vi "Analog Scan.vi"() -> ()   [LabVIEW 2020]
uses:
  Serial Support VISA.llb/Serial Actions.ctl
panel:
  out "He3/He4":dbl=0.027017159547280026 format="%.3f"
  out "Update":bool
  out "Total Pressure":dbl=1.3867864864864864e-05 format="%.3e"
  in  "stop":bool
  out "?":dbl[](graph)=[6.383227176220806e-09, 5.799363057324841e-09, 6.292993630573249e-09, 1.071751592356688e-07, 2.781942675159236e-07, 2.2762632696390657e-07, 3.148853503184713e-07, 4.156592356687898e-07, 5.076602972399151e-07, 5.451220806794055e-07, 5.554108280254777e-07, 5.598842887473461e-07, 4.985690021231423e-07, 3.8966985138004246e-07, 2.408577494692144e-07, 6.305732484076434e-08, 1.80552016985138e-08, 7.371549893842887e-09, 4.512738853503184e-09, 1.0222929936305733e-09, 3.142250530785562e-10, -1.8397027600849257e-09, 1.2845010615711252e-09, 8.70488322717622e-11, 2.2123142250530784e-09, 1.4118895966029723e-09, 4.543524416135881e-10, 5.165605095541402e-09, 8.238853503184713e-09, 1.0167728237791932e-08, 1.1630573248407643e-08, 1.0235668789808917e-08, 1.1387473460721868e-08, 9.991507430997877e-09, 5.780254777070063e-09, 1.959660297239915e-09, -9.851380042462845e-10, 3.7261146496815285e-10, -1.3237791932059447e-09, -5.6263269639065816e-11, -5.679405520169851e-10, -2.227176220806794e-09, 1.0042462845010616e-09, 8.938428874734607e-10, 7.91932059447983e-10, 4.447983014861995e-10, -1.4904458598726114e-09, 2.8662420382165604e-11, 2.083864118895966e-09, -3.5244161358811037e-10, -6.295116772823779e-10, -1.898089171974522e-09, 4.5010615711252653e-10, 1.9479830148619957e-09, -2.210191082802548e-09, 1.7908704883227175e-09, -6.114649681528662e-10, 7.027600849256899e-10, 2.2154989384288745e-09, -2.2367303609341826e-09, 3.5138004246284497e-10, -1.6475583864118898e-09, -1.2420382165605095e-09, 1.8004246284501061e-09, -2.4532908704883226e-09, -4.670912951167728e-11, -2.91932059447983e-10, 1.2738853503184715e-11, 2.489384288747346e-09, -2.265392781316348e-09, 8.439490445859872e-10, -3.354564755838641e-10, -7.526539278131635e-10, 2.421443736730361e-09, -2.700636942675159e-09, 9.861995753715497e-10, -7.887473460721868e-10, -6.157112526539278e-11, 2.832271762208068e-09, -2.252653927813163e-09, 2.62208067940552e-10, 2.1231422505307854e-11, -9.002123142250531e-10, 2.468152866242038e-09, -3.5360934182590233e-09, 8.386411889596603e-10, -5.870488322717621e-10, -3.927813163481953e-11, 2.1687898089171975e-09, -2.6104033970276008e-09, 7.282377919320594e-10, -6.900212314225053e-11, -1.2983014861995753e-09, 1.3832271762208068e-09, -2.6008492569002124e-09, 2.6751592356687895e-10, -5.870488322717621e-10, -2.7388535031847135e-10, 1.8630573248407644e-09, -2.178343949044586e-09, 8.397027600849257e-10, 4.978768577494691e-10, -2.218683651804671e-10, 1.7070063694267515e-09, -1.96072186836518e-09, 3.90552016985138e-09, 5.8046709129511675e-09, 6.473460721868365e-09, 9.766454352441613e-09, 9.27176220806794e-09, 1.16932059447983e-08, 1.3043524416135881e-08, 9.373673036093419e-09, 8.456475583864119e-09, 6.231422505307855e-10, 1.718683651804671e-09, 1.1464968152866242e-10, 1.3322717622080678e-09, 3.2547770700636943e-09, 1.054140127388535e-09, 4.818471337579618e-09, 4.9808917197452225e-09, 3.5e-09, 7.670912951167728e-09, 1.2777070063694267e-08, 5.751273885350318e-08, 1.5892462845010614e-07, 2.25776008492569e-07, 2.7426857749469213e-07, 3.0801380042462845e-07, 3.070297239915074e-07, 2.9790233545647557e-07, 2.338673036093418e-07, 1.5005626326963905e-07, 4.046815286624204e-08, 1.6974522292993628e-08, 1.4698513800424627e-08, 1.4262208067940551e-08, 1.869532908704883e-08, 1.897452229299363e-08, 2.06104033970276e-08, 2.2679405520169852e-08, 1.8743099787685772e-08, 1.7830148619957538e-08, 1.4470276008492568e-08, 3.696072186836518e-08, 8.625265392781315e-08, 1.211496815286624e-07, 1.4909235668789808e-07, 1.649692144373673e-07, 1.6709235668789808e-07, 1.6360828025477706e-07, 1.2956581740976644e-07, 8.94384288747346e-08, 4.8571125265392775e-08, 1.1504458598726114e-07, 2.6974734607218685e-07, 3.562579617834395e-07, 4.158556263269639e-07, 4.545021231422505e-07, 4.449851380042463e-07, 4.240583864118896e-07, 3.339023354564756e-07, 2.2270276008492568e-07, 1.6168895966029725e-07, 5.474246284501061e-07, 1.1831061571125264e-06, 1.4687940552016984e-06, 1.6797356687898089e-06, 1.7986709129511676e-06, 1.7556889596602972e-06, 1.5903195329087047e-06, 1.2338619957537154e-06, 6.22692144373673e-07, 7.33864118895966e-08, 2.1935244161358813e-08, 1.1503184713375797e-08, 4.5902335456475585e-09, 6.038216560509554e-09, 3.182590233545647e-09, 5.26963906581741e-09, 6.270700636942675e-09, 1.559447983014862e-09, 4.739915074309979e-09, 9.617834394904458e-10, 2.8959660297239915e-09, 8.386411889596603e-09, 7.348195329087049e-09, 1.187579617834395e-08, 1.1885350318471336e-08, 1.2576433121019108e-08, 1.345859872611465e-08, 8.524416135881104e-09, 7.46072186836518e-09, 8.768577494692145e-10, 2.4309978768577495e-10, 1.8290870488322718e-09, -2.3099787685774946e-09, 2.0021231422505306e-09, 4.660297239915074e-10, -3.131634819532909e-10, 2.663481953290871e-09, -3.268577494692144e-09, 2.9670912951167727e-09, -6.624203821656051e-10, -2.4203821656050955e-10, 1.887473460721868e-09, -3.3832271762208065e-09, 2.900212314225053e-09, 1.0987261146496815e-09, 4.214437367303609e-10, 3.409766454352441e-09, -3.73036093418259e-09, 3.347133757961783e-09, 2.5477707006369425e-10, -4.830148619957538e-10, 1.3513800424628452e-09, -3.3726114649681525e-09, 2.726114649681529e-09, -7.399150743099787e-10, -4.851380042462844e-10, 8.853503184713376e-10, -3.8343949044585986e-09, 1.6560509554140127e-09, 1.4225053078556263e-10, 3.322717622080679e-10, 2.346072186836518e-09, -1.592356687898089e-09, 2.0668789808917195e-09, -2.8662420382165605e-10, -9.978768577494691e-11, 1.8227176220806794e-09, -1.6581740976645436e-09, 7.112526539278132e-10, 6.581740976645435e-11, -3.8641188959660294e-10, 2.4989384288747344e-09, -2.1125265392781315e-10, 3.805732484076433e-09, 2.859872611464968e-09, 7.346072186836518e-10, 3.2749469214437367e-09, -3.036093418259023e-10, 2.809978768577495e-09, 1.548832271762208e-09, 1.6624203821656051e-09, 7.0552016985138e-09, 6.6390658174097665e-09, 1.0763269639065816e-08, 1.2296178343949044e-08, 1.1033970276008492e-08, 1.2984076433121018e-08, 8.621019108280254e-09, 8.61995753715499e-09, 6.9150743099787685e-09, 7.855626326963907e-09, 1.7604033970276007e-08, 2.3303609341825902e-08, 3.431422505307855e-08, 4.2420382165605094e-08, 4.5386411889596607e-08, 5.847876857749469e-08, 7.803397027600848e-08, 1.6784713375796176e-07, 6.971645435244161e-07, 1.7668067940552016e-06, 3.019504246284501e-06, 3.886766454352441e-06, 4.702408704883227e-06, 4.463633757961783e-06, 4.6100265392781315e-06, 3.718911889596603e-06, 2.791633757961783e-06, 8.391847133757962e-07, 8.05392781316348e-08, 3.50859872611465e-08, 4.0593418259023356e-08, 5.079617834394904e-08, 6.51104033970276e-08, 7.172186836518046e-08, 6.781104033970276e-08, 6.857430997876858e-08, 5.394055201698514e-08, 3.683227176220807e-08, 2.2660297239915072e-08, 2.6995753715498938e-08, 5.3130573248407646e-08, 7.126220806794055e-08, 9.040976645435244e-08, 9.529405520169851e-08, 8.868683651804669e-08, 8.872505307855626e-08, 6.970488322717622e-08, 4.276220806794055e-08, 1.628980891719745e-08, 4.8481953290870486e-09, 6.028662420382165e-09, 4.618895966029724e-09, 5.816348195329087e-09, 7.039278131634819e-09, 4.803609341825902e-09, 1.0790870488322717e-08, 1.55e-08, 3.859766454352442e-08, 1.5550212314225054e-07, 3.73036093418259e-07, 6.452929936305732e-07, 8.339670912951168e-07, 1.02126008492569e-06, 9.69104033970276e-07, 9.633386411889595e-07, 7.602579617834394e-07, 5.648811040339703e-07, 1.7700849256900214e-07, 3.628768577494692e-08, 1.0143312101910827e-08, 6.323779193205945e-09, 2.2738853503184712e-09, 1.6337579617834394e-09, 2.8152866242038216e-09, -7.346072186836518e-10, 4.664543524416136e-09, 3.81104033970276e-10, 9.777070063694266e-10, 1.602972399150743e-09, 3.7367303609341825e-10, 4.490445859872611e-09, 3.571125265392781e-09, 3.9851380042462845e-09, 6.23248407643312e-09, 2.733545647558386e-09, 5.329087048832271e-09, 3.6019108280254775e-09, 7.08067940552017e-10, 1.6019108280254778e-09, -2.872611464968153e-09, 2.812101910828025e-09, -5.350318471337579e-10, -7.399150743099787e-10, 1.618895966029724e-09, -1.089171974522293e-09, 3.186836518046709e-09, 1.2261146496815287e-09, -1.3906581740976646e-10, 1.2420382165605095e-09, -2.0254777070063695e-09, 4.4575371549893845e-09, 2.9171974522292996e-09, 1.7675159235668788e-09, 4.549893842887473e-09, 1.562632696390658e-09, 4.574309978768578e-09, 2.7091295116772822e-09, -1.4331210191082802e-10, 1.0690021231422503e-09, -1.1624203821656052e-09, 3.929936305732484e-09, 1.6146496815286623e-09, 5.5201698513800425e-11, 2.208067940552017e-09, 1.6337579617834394e-09, 1.478768577494692e-09, 2.356687898089172e-09, 1.915074309978769e-09, -3.7898089171974525e-10, -2.673036093418259e-09, 6.7038216560509555e-09, 3.6985138004246285e-09, 8.619957537154989e-10, 6.666666666666666e-09, 3.019108280254777e-09, 4.492569002123142e-09, 5.253715498938428e-09, 1.0297239915074311e-10, 4.4405520169851374e-09, 4.580679405520169e-09, 9.042462845010616e-09, 1.1280254777070063e-08, 1.4046709129511675e-08, 1.9788747346072187e-08, 1.8685774946921442e-08, 2.0116772823779194e-08, 1.632271762208068e-08, 1.4576433121019106e-08, 2.1111464968152864e-08, 3.171656050955414e-08, 5.061783439490446e-08, 6.678025477707007e-08, 8.203078556263269e-08, 8.868895966029723e-08, 8.308811040339703e-08, 7.016985138004246e-08, 4.989596602972399e-08, 2.2325902335456473e-08, 1.228343949044586e-08, 1.010828025477707e-08, 1.61380042462845e-08, 2.1570063694267515e-08, 2.638535031847134e-08, 3.4994692144373673e-08, 3.454246284501062e-08, 3.357749469214437e-08, 2.6528662420382164e-08, 1.7306794055201698e-08, 1.0711252653927812e-08, 6.645435244161359e-09, 7.955414012738853e-09, 1.0701698513800425e-08, 1.2320594479830148e-08, 1.7985138004246285e-08, 1.778343949044586e-08, 1.764012738853503e-08, 1.4130573248407644e-08, 9.255838641188959e-09, 9.613588110403396e-09, 1.0737791932059447e-08, 1.76932059447983e-08, 2.5336518046709128e-08, 3.173566878980892e-08, 4.130042462845011e-08, 4.196815286624204e-08, 4.0684713375796174e-08, 3.383227176220807e-08, 2.62484076433121e-08, 2.997133757961783e-08, 4.221974522292994e-08, 6.70552016985138e-08, 9.160721868365181e-08, 1.143832271762208e-07, 1.3030891719745224e-07, 1.271963906581741e-07, 1.0675265392781316e-07, 7.839808917197452e-08, 4.0634819532908706e-08, 1.7104033970276006e-08, 7.511677282377919e-09, 5.953290870488322e-09, 6.330148619957537e-09, 6.634819532908705e-09, 1.0242038216560509e-08, 9.682590233545646e-09, 9.025477707006369e-09, 7.389596602972399e-09, 3.789808917197452e-09, 3.0053078556263266e-09, 2.770700636942675e-10, -4.214437367303609e-10, 1.870488322717622e-09, 2.4235668789808915e-09, 3.557324840764331e-09, 1.9819532908704882e-09, 1.6613588110403397e-09, 1.8715498938428875e-09, 1.6687898089171974e-09, -4.777070063694267e-11, 1.2558386411889594e-09, -1.2399150743099786e-09, 1.3853503184713377e-09, 1.4331210191082802e-09, 1.0881104033970277e-09, -3.290870488322717e-11, -5.955414012738853e-10, 3.418259023354565e-10, -7.441613588110403e-10, 1.8726114649681527e-09, -2.2611464968152866e-10, -6.061571125265393e-10, 1.3375796178343947e-10, 9.320594479830148e-10, -7.547770700636943e-10, 1.1624203821656052e-09, -1.7038216560509556e-09, 5.732484076433121e-11, 1.6889596602972398e-09, 1.1815286624203822e-09, -1.9532908704883225e-10, -1.2303609341825903e-09, 3.9808917197452225e-10, 1.708067940552017e-09, -4.968152866242038e-10, 9.288747346072187e-10, -1.0116772823779193e-09, 2.1231422505307857e-12, 3.21656050955414e-10, 1.0403397027600848e-09, 6.878980891719745e-10, -1.516985138004246e-09, 2.043524416135881e-09, 3.3046709129511675e-09, 3.0774946921443734e-09, 2.2749469214437365e-09]
  out "Steps/AMU":dbl=10.0 format="%.2f"
  out "Final Mass":dbl=50.0 format="%.2f"
  out "Initial Mass":dbl=1.0 format="%.2f"
  out "Partial Pressure\nSensitivity Factor":dbl=0.0942 format="%.2f"
  out "Number of Points":u32=491
  in  "Port Number":refnum<visa-resource-name>="ASRL1::INSTR"
  in  "error in (no error)":errorcluster
  in  "Timeout Limit":dbl=20.0 format="%.2f"
  out "error out":errorcluster
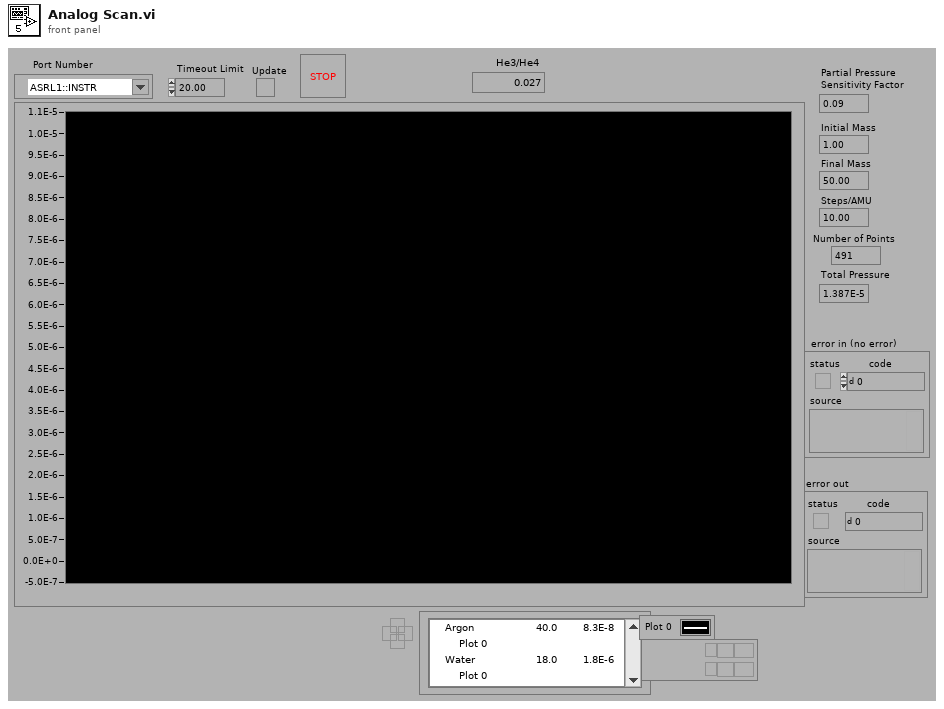
[diagram p1: front panel]
types:
  T1 = cluster{"Number of Points":u32, "Initial Mass":dbl, "Final Mass":dbl, "Steps/AMU":dbl, "Partial Pressure\nSensitivity Factor":dbl}
  T2 = typedef "Serial Actions.ctl" = enum16{"Init", "Break", "Clear Buffer", "Write", "Read", "N Bytes", "Lock", "Unlock", "Close"}
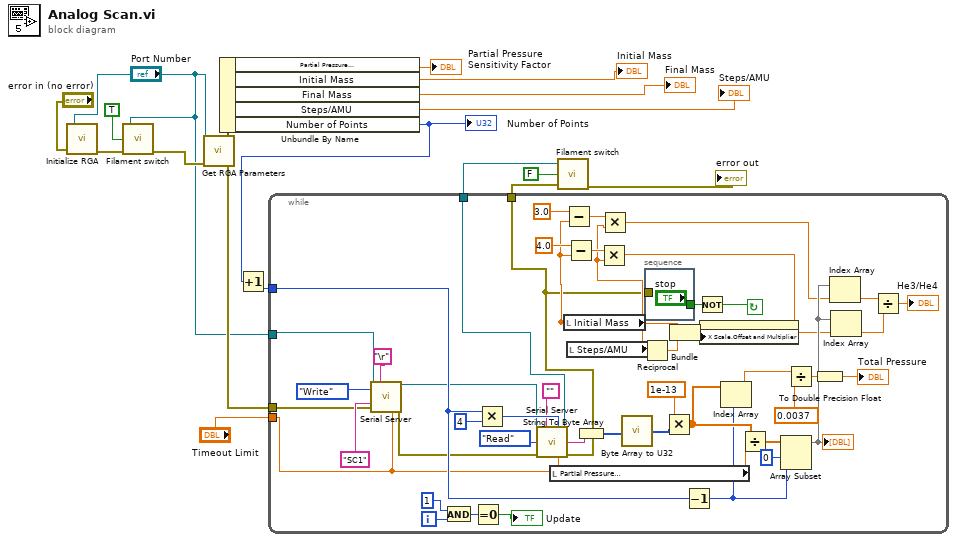
[diagram p0: block diagram]
diagram:
  n1 = call "Initialize RGA.vi"("Port Number"="Port Number", "error in (no error)"="error in (no error)") -> ("error out"=w8:errorcluster)  [unwired: 1 in, 3 out]
  n2 = call "Filament switch.vi"("Port Number"="Port Number", "Filament Switch"=TRUE, "error in (no error)"=w8) -> ("error out"=w7:errorcluster)  [unwired: 3 out]
  n3 = call "Get RGA Parameters.vi"("Port Number"="Port Number", "error in (no error)"=w7) -> ("RGA Parameters"=w17:T1, "error out"=w10:errorcluster)  [unwired: 1 in]
  n4 = Unbundle By Name(w17) -> ("Partial Pressure\nSensitivity Factor"=→"Partial Pressure\nSensitivity Factor":dbl, "Initial Mass"=→"Initial Mass":dbl, "Final Mass"=→"Final Mass":dbl, "Steps/AMU"=→"Steps/AMU":dbl, "Number of Points"=w12:u32)
  "Number of Points" <- w12
  n5 = Increment(x=w12) -> (x+1=w18:u32)
  n6 = while {
    tunnel: [w19] -> w2
    tunnel: [w20] -> w4
    tunnel: w10 -> [w38]
    tunnel: w18 -> [w50]
    tunnel: "Timeout Limit" -> [w36]
    tunnel: "Port Number" -> [w22]
    i -> [w45]
    stop <- w64 continue-if-true
    n7 = call "Serial Server.vi"("VISA Resource Name"=w22, "EOT Chars (cr/lf)"="\r", "Action"=Serial_Actions."Write", "String To Send"="SC1", "error in (no error)"=w38, "Timeout Limit(sec)"=w36) -> ("dup VISA Resource Name"=w21:refnum<visa-resource-name>, "error out"=w37:errorcluster)  [unwired: 5 in, 3 out]
    n8 = And(x=1, y=w45) -> (x .and. y?=w43:i32)
    n9 = Equal To 0?(x=w43) -> (x = 0?=→"Update":bool)
    n10 = Multiply(x=w50, y=4) -> (x*y=w60:u32)
    n11 = call "Serial Server.vi"("VISA Resource Name"=w21, "EOT Chars (cr/lf)"="", "Max Char to Read"=w60, "Action"=Serial_Actions."Read", "error in (no error)"=w37, "Timeout Limit(sec)"=w36) -> ("dup VISA Resource Name"=w20:refnum<visa-resource-name>, "Serial Read"=w59:string, "error out"=w19:errorcluster)  [unwired: 5 in, 2 out]
    n12 = local read "Partial Pressure\nSensitivity Factor"() -> (w56:dbl)
    n13 = local read "Initial Mass"() -> (w29:dbl)
    n14 = Subtract(x=3.0 ("y"), y=w29) -> (x-y=w28:dbl)
    n15 = Subtract(x=4.0 ("y"), y=w29) -> (x-y=w27:dbl)
    n16 = local read "Steps/AMU"() -> (w26:dbl)
    n17 = String To Byte Array(string=w59) -> (unsigned byte array=w58:u8[])
    n18 = Multiply(x=w27, y=w26) -> (x*y=w24:dbl)
    n19 = Multiply(x=w28, y=w26) -> (x*y=w25:dbl)
    n20 = call "Byte Array to U32.vi"("Input Bytes"=w58) -> ("Output Integers"=w55:i32[])
    n21 = Reciprocal(x=w26) -> (1/x=w52:dbl)
    n22 = stacked-sequence {
      tunnel: ["stop"] -> w65
      tunnel: w19 -> [_]
      frame #0 {
      }
    }
    n23 = Multiply(x=1e-13, y=w55) -> (x*y=w49:dbl[])
    n24 = Bundle("Initial Mass"=w29, w52) -> (w51:cluster{"Initial Mass":dbl, dbl})  [unwired: 1 in]
    n25 = Decrement(x=w50) -> (x-1=w48:u32)
    n26 = Not(x=w65) -> (.not. x?=w64:bool)
    n27 = property class="WFGraph (strict)"("X Scale.Offset and Multiplier"=w51) -> ()  [unwired: 2 in, 2 out]
    n28 = Index Array(array=w49, index=w48) -> (element=w47:dbl)
    n29 = Divide(x=w49, y=w56) -> (x/y=w54:dbl[])
    n30 = Array Subset(array=w54, index=0, length=w48) -> (w35:dbl[])
    "?" <- w35
    n31 = Divide(x=w47, y=0.0037) -> (x/y=w63:dbl)
    n32 = To Double Precision Float(number=w63) -> (double precision float=→"Total Pressure":dbl)
    n33 = Index Array(array=w35, index=w25) -> (element=w34:dbl)
    n34 = Index Array(array=w35, index=w24) -> (element=w33:dbl)
    n35 = Divide(x=w34, y=w33) -> (x/y=→"He3/He4":dbl)
  }
  n36 = call "Filament switch.vi"("Port Number"=w4, "Filament Switch"=FALSE, "error in (no error)"=w2) -> ("error out"=→"error out":errorcluster)  [unwired: 3 out]
